vi "Init.vi"(5 "CS":refnum<class "SPI CS.lvclass">, 7 "SPI":refnum<class "SPI.lvclass">, 8 "error in (no error)":errorcluster) -> (0 "error out":errorcluster, 3 "SPI Device out":refnum<class "SPI Device.lvclass">)   [LabVIEW 2020, in "CTI.lvlib" / "SPI Device.lvclass"]
uses:
  SPI Device.lvclass
  SPI Device.lvclass/SPI Device.ctl
  SPI/SPI.lvclass
  SPI CS/SPI CS.lvclass
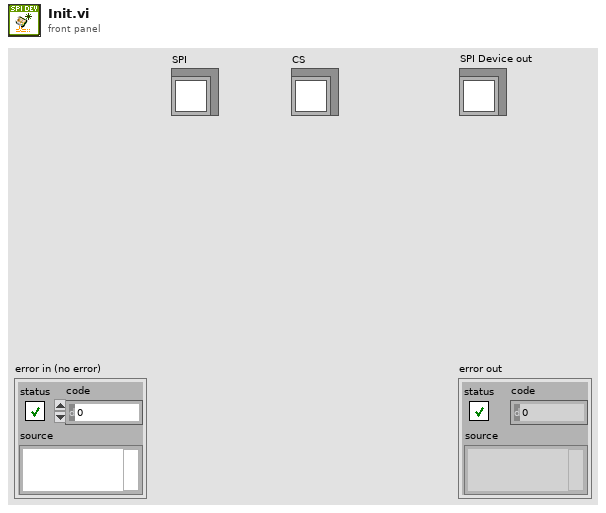
[diagram p1: front panel]
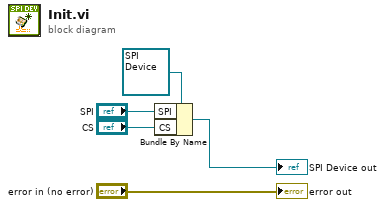
[diagram p0: block diagram]
diagram:
  n1 = Bundle By Name(cluster=refnum<class "SPI Device.lvclass"> refnum ("SPI Device in"), "SPI"="SPI", "CS"="CS") -> (→"SPI Device out":refnum<class "SPI Device.lvclass">)
  "error out" <- "error in (no error)"
